vi "Teleop.vi"(10 "Match Info":T1={"Autonomous Elapsed Seconds"=0.0, "TeleOp Elapsed Seconds"=0.0, "Disabled Elapsed Seconds"=0.0, "Visited Autonomous"=FALSE, "Visited TeleOp"=FALSE, "Visited Disabled"=FALSE, "Autonomous Settings"={"Autonomous Style"=enum."Independent", "VI Refnum"=refnum}}, 11 "Call Context":T2) -> ()   [LabVIEW 2017]
doc: "This VI is called for each enabled TeleOp packet received from the DS. It is typically used to read from joysticks and other inputs and update I/O or setpoints for timed control loops. It should complete and return within 20 milliseconds or risk missing DS packets."
uses:
  <vilib>/Rock Robotics/WPI/DriverStation/WPI_DriverStationDerivedRobotMode.ctl
  <vilib>/Rock Robotics/WPI/DriverStation/WPI_DriverStationMatch Info.ctl
  <vilib>/Rock Robotics/WPI/Utilities/WPI_GetSetVariantRefNum.vi
panel:
  out "f 2":dbl
  out "f":dbl
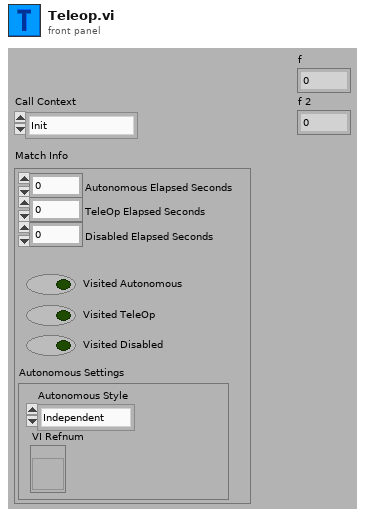
[diagram p1: front panel]
types:
  T1 = typedef "WPI_DriverStationMatch Info.ctl" = cluster{"Autonomous Elapsed Seconds":dbl, "TeleOp Elapsed Seconds":dbl, "Disabled Elapsed Seconds":dbl, "Visited Autonomous":bool, "Visited TeleOp":bool, "Visited Disabled":bool, "Autonomous Settings":cluster{"Autonomous Style":enum16{"Iterative", "Independent"}, "VI Refnum":refnum<vi>}}
  T2 = typedef "WPI_DriverStationDerivedRobotMode.ctl" = enum16{"Init", "Execute", "Stop"}
  T3 = typedef "WPI_JoystickDevRef.ctl" = cluster{"Device":T4}
  T4 = typedef "WPI_JoystickDeviceEnum.ctl" = enum16{"USB 0", "USB 1", "USB 2", "USB 3", "USB 4", "USB 5"}
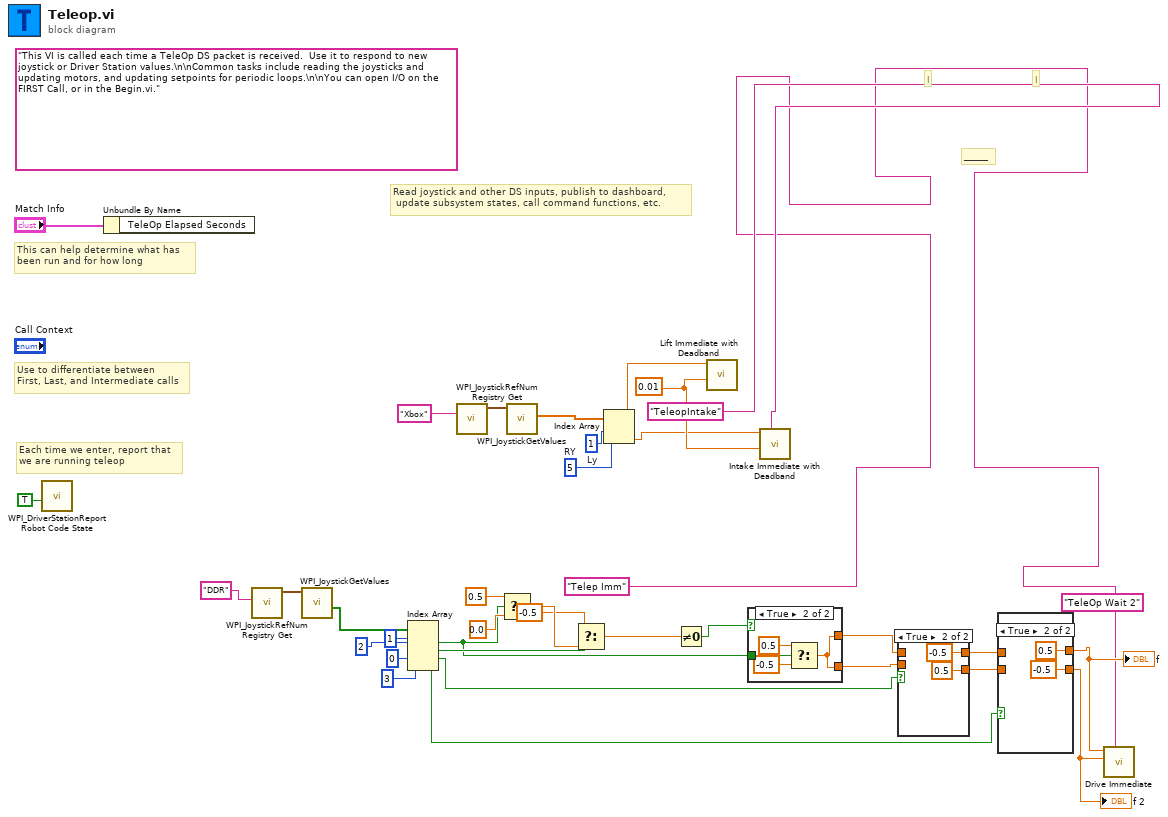
[diagram p0: block diagram]
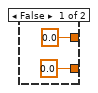
[diagram p4: hidden frame]
diagram:
  w28 = 5  # RY
  w29 = 1  # Ly
  w30 = 0.01 ("Deadband Value")
  (unwired) "TeleOp Wait 2" ("Description")
  (unwired) "This VI is called each time a TeleOp DS packet is received.  Use it to respond to new joystick or Driver Station values.\n\nCommon tasks include reading the joysticks and updating motors, and updating setpoints for periodic loops.\n\nYou can open I/O on the FIRST Call, or in the Begin.vi."
  # "|"
  # "|"
  # "______"
  # "Read joystick and other DS inputs, publish to dashboard,\n update subsystem states, call command functions, etc."
  # "Each time we enter, report that\nwe are running teleop"
  # "Use to differentiate between\nFirst, Last, and Intermediate calls"
  # "This can help determine what has\nbeen run and for how long"
  n1 = call <vilib>:"WPI_DriverStationReport Robot Code State.vi"("TeleOp"=TRUE ("Autonomous")) -> ()  [unwired: 10 in, 1 out]
  n2 = Unbundle By Name("Match Info") -> ()  [unwired: 1 out]
  n3 = call <vilib>:"WPI_JoystickRefNum Registry Get.vi"("refnum name"="DDR") -> ("JoystickDevRef"=w24:T3)  [unwired: 1 in, 9 out]
  n4 = call <vilib>:"WPI_JoystickGetValues.vi"("JoystickDevRef"=w24) -> ("Buttons"=w23:bool[])  [unwired: 6 in, 4 out]
  n5 = Index Array(array=w23, index #1=2 ("index"), index #2=1 ("index"), index #3=0 ("index"), index #4=3 ("index")) -> (element #1=w3:bool, element #2=w18:bool, element #3=w9:bool, element #4=w4:bool)
  n6 = call <vilib>:"WPI_JoystickRefNum Registry Get.vi"("refnum name"="Xbox") -> ("JoystickDevRef"=w32:T3)  [unwired: 1 in, 9 out]
  n7 = Select(t=0.5, s=w3, f=0.0) -> (s? t:f=w15:dbl)
  n8 = call <vilib>:"WPI_JoystickGetValues.vi"("JoystickDevRef"=w32) -> ("Axes"=w31:dbl[])  [unwired: 6 in, 4 out]
  n9 = Select(t=-0.5, s=w18, f=w15) -> (s? t:f=w12:dbl)
  n10 = Index Array(array=w31, index #1=w29, index #2=w28) -> (element #1=w27:dbl, element #2=w26:dbl)
  n11 = Not Equal To 0?(x=w12) -> (x != 0?=w13:bool)
  n12 = call "Lift Immediate with Deadband.vi"("Deadband Value"=w30, "Setpoint"=w27) -> ()  [unwired: 9 in, 1 out]
  n13 = case shown="True" w13 {
    tunnel: [0.0 w39] -> w10
    tunnel: [0.0 w39] -> w11
    tunnel: w3 -> [_ w38]
    frame False {
    }
    frame True {
      n14 = Select(t=0.5, s=w38, f=-0.5) -> (s? t:f=w39:dbl)
    }
  }
  n15 = call "Intake Immediate with Deadband.vi"("Description"="TeleopIntake", "Deadband Value"=w30, "Setpoint"=w26) -> ()  [unwired: 8 in, 1 out]
  n16 = case shown="True" w9 {
    tunnel: w11 -> [w43 _]
    tunnel: w10 -> [w42 _]
    tunnel: [w43 -0.5 ("f")] -> w8
    tunnel: [w42 0.5 ("f")] -> w7
    frame False {
    }
    frame True {
    }
  }
  n17 = case shown="True" w4 {
    tunnel: w8 -> [w47 _]
    tunnel: w7 -> [w46 _]
    tunnel: [w47 0.5 ("f")] -> w5
    tunnel: [w46 -0.5 ("f")] -> w6
    frame False {
    }
    frame True {
    }
  }
  "f" <- w5
  "f 2" <- w6
  n18 = call "Drive Immediate.vi"("Description"="Telep Imm", "Right Setpoint"=w6, "Left Setpoint"=w5) -> ()  [unwired: 8 in, 1 out]
